vi "Main Page.vi"(8 "error in (no error)":errorcluster, 11 "Node Ptr":T1 format="%.0x") -> (0 "error out":errorcluster)   [LabVIEW 2019, in "DeltaPSControl System Explorer.lvlib"]
uses:
  DeltaPSControl System Explorer.lvlib
  <vilib>/NI VeriStand/Custom Device API/Custom Device Item Ref.ctl
  Shared/Constants.vi
  <vilib>/NI VeriStand/Custom Device API/Get Item Property (String).vi
  <vilib>/NI VeriStand/Custom Device API/Get Item Property (U16).vi
  <vilib>/NI VeriStand/Custom Device API/Get Item Property (String Array).vi
  <vilib>/NI VeriStand/Custom Device API/Set Item Property (String).vi
  <vilib>/NI VeriStand/Custom Device API/Set Item Property (U16).vi
  <vilib>/NI VeriStand/Custom Device API/Set Item Property (String Array).vi
  <vilib>/NI VeriStand/Custom Device API/Custom Device API.lvlib
  Shared/DeltaPSControl Shared.lvlib
panel:
  in  "Help":bool
  out "Sequences List":string[][](array[string])
  in  "LOAD Seq":bool
  in  "Port":u16
  in  "IP Address":string
  in  "Header":cluster{"Section Name":string}={"Section Name"="Custom Device Item Settings"}
  in  "Description":string
  in  "Name":string
  # "Always need to load\n sequences,\n to be able to use them."
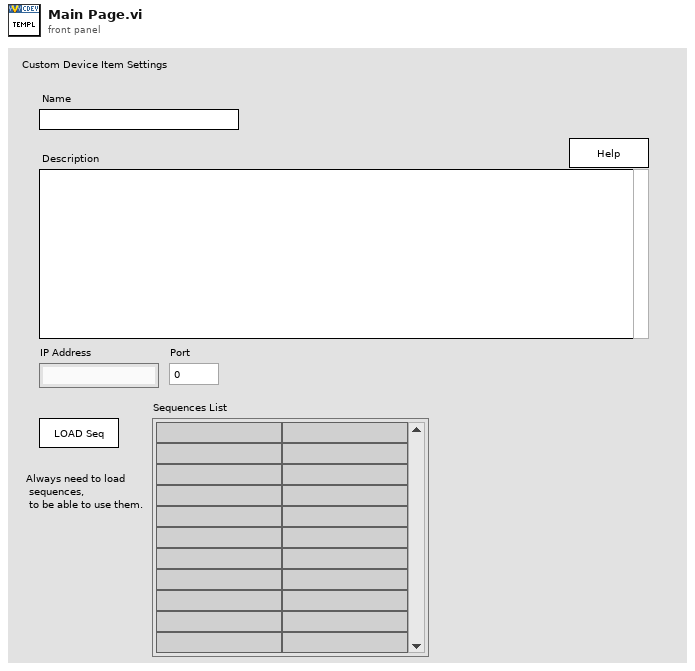
[diagram p1: front panel]
types:
  T1 = typedef "Custom Device API.lvlib/Custom Device Item Ref.ctl" = u64
  T2 = typedef "Custom Device API.lvlib/Custom Device Item Info.ctl" = cluster{"Name":string, "Is Channel":bool, "GUID":string, "Is Waveform":bool}
  T3 = typedef "Custom Device API.lvlib/Custom Device Commands.ctl" = enum16{"Default", "Item renamed", "Shutdown", "Dynamic button pressed"}
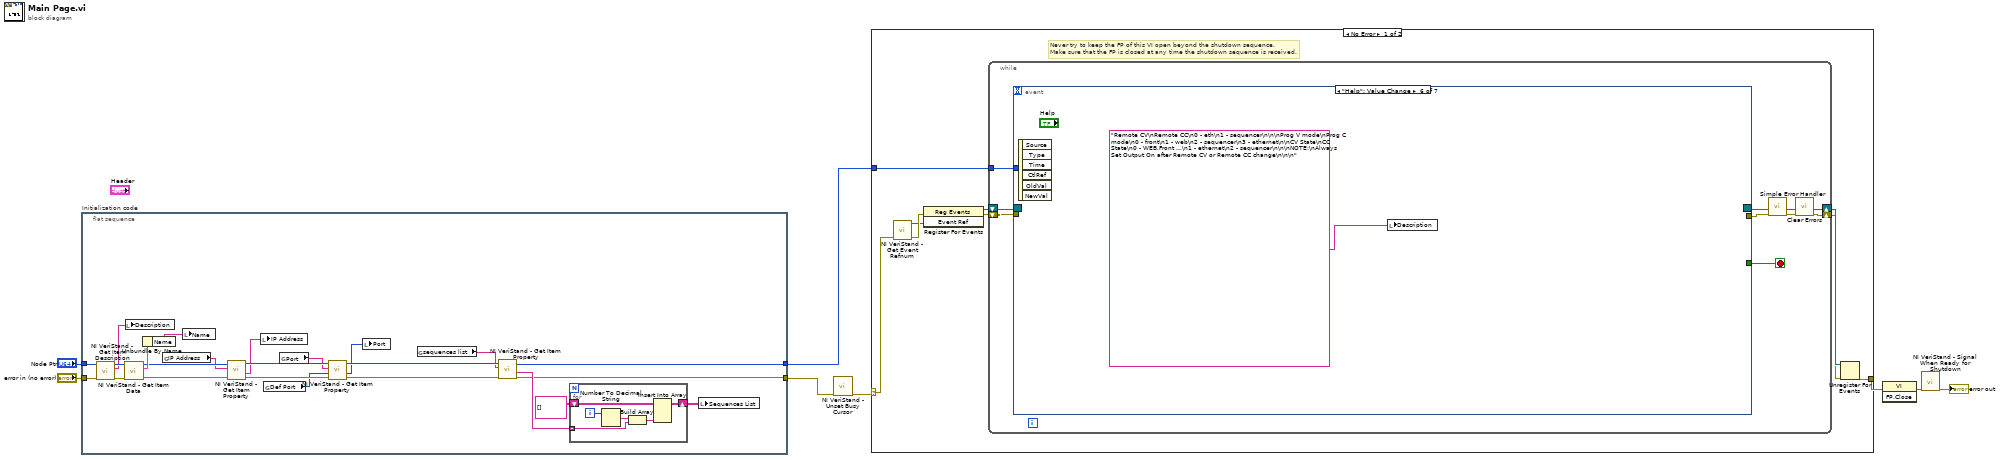
[diagram p0: block diagram]
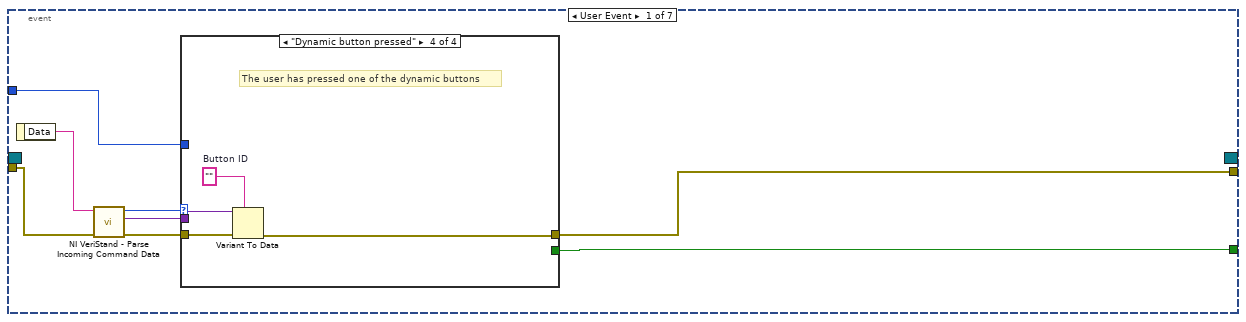
[diagram p2: hidden frame]
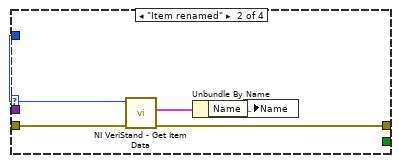
[diagram p4: hidden frame]
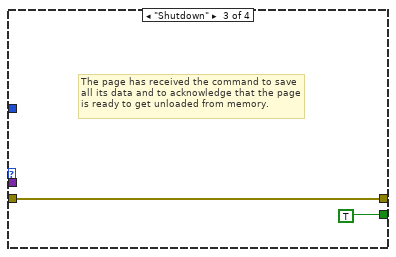
[diagram p5: hidden frame]
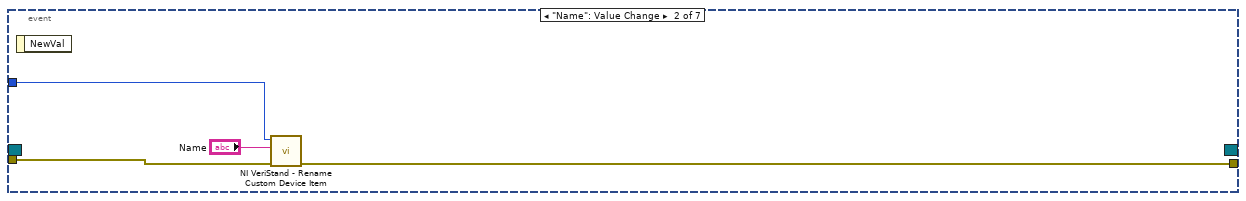
[diagram p6: hidden frame]
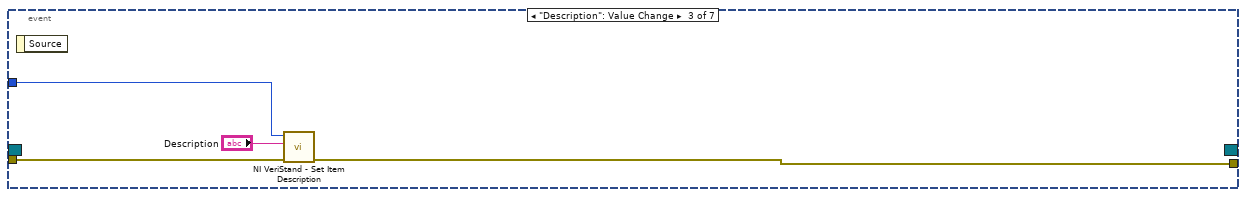
[diagram p7: hidden frame]
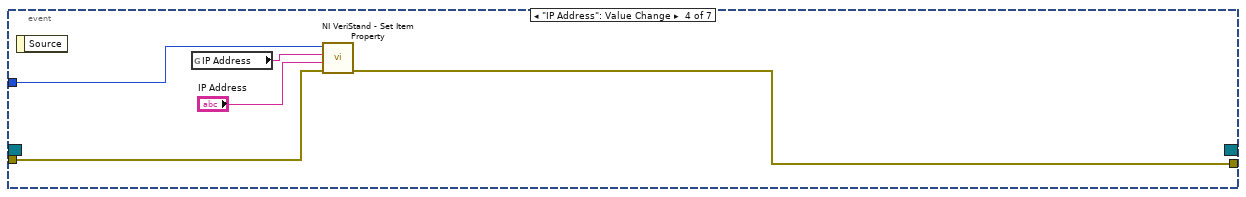
[diagram p8: hidden frame]
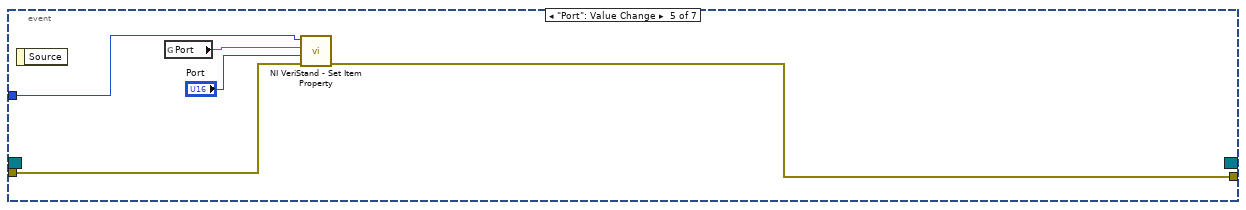
[diagram p9: hidden frame]
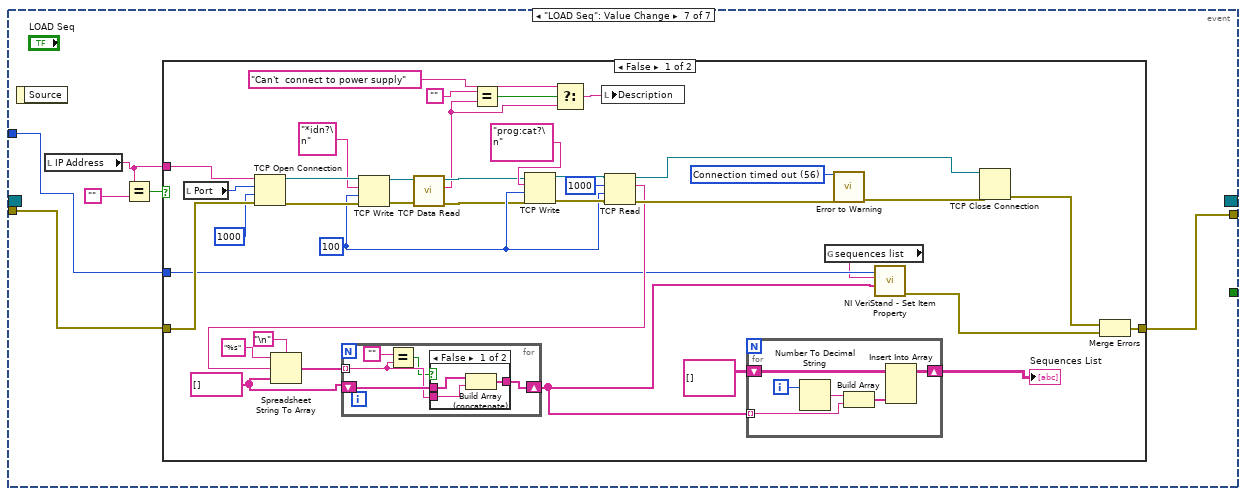
[diagram p10: hidden frame]
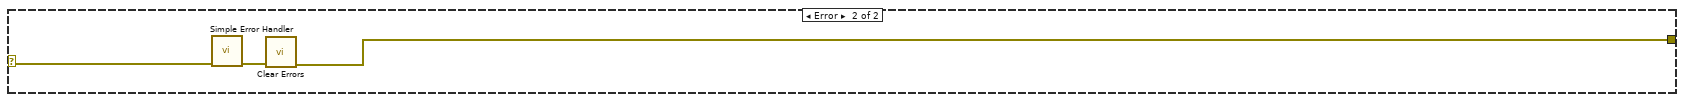
[diagram p13: hidden frame]
diagram:
  n1 = flat-sequence "Initialization code" {
    tunnel: "error in (no error)" -> [w31]
    tunnel: "Node Ptr" -> [w30]
    tunnel: [w16] -> w4
    tunnel: [w17] -> w1
    frame #0 {
      n2 = call <vilib>:"NI VeriStand - Get Item Description.vi"("error in (no error)"=w31, "Item Ref in"=w30) -> ("error out"=w28:errorcluster, "Description"=w29:string, "Item Ref out"=w32:T1)  [unwired: 7 out]
      n3 = call <vilib>:"NI VeriStand - Get Item Data.vi"("error in (no error)"=w28, "Item Ref in"=w32) -> ("error out"=w18:errorcluster, "Item Info"=w27:T2, "Item Ref out"=w19:T1)  [unwired: 7 out]
      n4 = local write "Description"(w29) -> ()
      n5 = Unbundle By Name(w27) -> ("Name"=w26:string)
      n6 = global read "Constants.vi" "IP Address"() -> (w12:string)
      n7 = local write "Name"(w26) -> ()
      n8 = call-poly <vilib>:"NI VeriStand - Get Item Property.vi"("error in (no error)"=w18, "Property Name"=w12, "Item Ref in"=w19) -> ("error out"=w21:errorcluster, "Value"=w15:string, "Item Ref out"=w22:T1)  [unwired: 5 in, 1 out]
      n9 = local write "IP Address"(w15) -> ()
      n10 = global read "Constants.vi" "Def Port"() -> (w9:u16)
      n11 = global read "Constants.vi" "Port"() -> (w11:string)
      n12 = call-poly <vilib>:"NI VeriStand - Get Item Property.vi"("error in (no error)"=w21, "Default Value"=w9, "Property Name"=w11, "Item Ref in"=w22) -> ("error out"=w23:errorcluster, "Value"=w14:u16, "Item Ref out"=w24:T1)  [unwired: 4 in, 1 out]
      n13 = local write "Port"(w14) -> ()
      n14 = global read "Constants.vi" "sequences list"() -> (w10:string)
      n15 = call-poly <vilib>:"NI VeriStand - Get Item Property.vi"("error in (no error)"=w23, "Property Name"=w10, "Item Ref in"=w24) -> ("error out"=w16:errorcluster, "Value"=w25:string[], "Item Ref out"=w17:T1)  [unwired: 5 in, 1 out]
      n16 = for {
        shift-right: [w37] -> w13
        shift-left: string[][] [] -> [w38]
        tunnel: w25 -> [w33] mode=indexing
        i -> [w36]
        n17 = Number To Decimal String(number=w36) -> (decimal integer string=w35:string)  [unwired: 1 in]
        n18 = Build Array(w35, w33) -> (w34:string[])
        n19 = Insert Into Array(array=w38, new element=w34) -> (w37:string[][])  [unwired: 2 in]
      }
      n20 = local write "Sequences List"(w13) -> ()
    }
  }
  n21 = call <vilib>:"NI VeriStand - Unset Busy Cursor.vi"("error in (no error)"=w4) -> ("error out"=w3:errorcluster)  [unwired: 10 out]
  n22 = case shown="No Error" w3 {
    selector: w3 -> [w39 w157]
    tunnel: [w44 w155] -> w8
    tunnel: w1 -> [w40 _]
    frame No Error {
      # "Never try to keep the FP of this VI open beyond the shutdown sequence.\nMake sure that the FP is closed at any time the shutdown sequence is received."
      n23 = call <vilib>:"NI VeriStand - Get Event Refnum.vi"("error in (no error)"=w39) -> ("error out"=w47:errorcluster, "Event Ref"=w43:refnum<user-event>)  [unwired: 9 out]
      n24 = register-events(error in=w47, w43) -> (reference out=w41:refnum<event-registration>, error out=w42:errorcluster)  [unwired: 1 in]
      n25 = while {
        tunnel: w40 -> [w51]
        shift-right: [w48] -> w45
        shift-left: w42 -> [w54]
        shift-right: [w55] -> w46
        shift-left: w41 -> [w53]
        stop <- w52 stop-if-true
        n26 = event shown="[5] \"Help\": Value Change" {
          selector: w53 -> [_ _ _ _ _ _ _]
          dyn-events: [_ _ _ _ _ _ _] -> w55
          timeout: _ -> [_ _ _ _ _ _ _]
          tunnel: w54 -> [w63 w79 w82 w86 w92 _ w96]
          tunnel: [w59 _ _ _ _ _ _] -> w52
          tunnel: [w58 w78 w81 w85 w91 _ w95] -> w50
          tunnel: w51 -> [w57 w77 w83 w87 w89 _ w97]
          event User Event {
            n27 = event-data() -> ("Data"=w62:string)  [unwired: 1 out]
            n28 = call <vilib>:"NI VeriStand - Parse Incoming Command Data.vi"("error in (no error)"=w63, "Incoming data"=w62) -> ("error out"=w61:errorcluster, "Outgoing data"=w56:variant, "Action"=w60:T3)  [unwired: 7 out]
            n29 = case shown="\"Dynamic button pressed\"" w60 {
              tunnel: w61 -> [w64 w69 w70 w75]
              tunnel: [_ _ TRUE _] -> w59
              tunnel: [w64 w66 w70 w72] -> w58
              tunnel: w57 -> [_ w68 _ _]
              tunnel: w56 -> [_ _ _ w74]
              frame "Default", Default {
              }
              frame "Item renamed" {
                n30 = call <vilib>:"NI VeriStand - Get Item Data.vi"("error in (no error)"=w69, "Item Ref in"=w68) -> ("error out"=w66:errorcluster, "Item Info"=w67:T2)  [unwired: 8 out]
                n31 = Unbundle By Name(w67) -> ("Name"=w65:string)
                n32 = local write "Name"(w65) -> ()
              }
              frame "Shutdown" {
                # "The page has received the command to save all its data and to acknowledge that the page is ready to get unloaded from memory."
              }
              frame "Dynamic button pressed" {
                w73 = ""  # Button ID
                # "The user has pressed one of the dynamic buttons"
                n33 = Variant To Data(error in=w75, type=w73, Variant=w74) -> (error out=w72:errorcluster)  [unwired: 1 out]
              }
            }
          }
          event "Name": Value Change {
            n34 = event-data() -> ()  [unwired: 2 out]
            n35 = call <vilib>:"NI VeriStand - Rename Custom Device Item.vi"("error in (no error)"=w79, "New Name"="Name", "Item Ref in"=w77) -> ("error out"=w78:errorcluster)  [unwired: 1 in, 7 out]
          }
          event "Description": Value Change {
            n36 = event-data() -> ()  [unwired: 2 out]
            n37 = call <vilib>:"NI VeriStand - Set Item Description.vi"("error in (no error)"=w82, "Description"="Description", "Item Ref in"=w83) -> ("error out"=w81:errorcluster)  [unwired: 8 out]
          }
          event "IP Address": Value Change {
            n38 = event-data() -> ()  [unwired: 2 out]
            n39 = global read "Constants.vi" "IP Address"() -> (w88:string)
            n40 = call-poly <vilib>:"NI VeriStand - Set Item Property.vi"("error in (no error)"=w86, "Value"="IP Address", "Property Name"=w88, "Item Ref in"=w87) -> ("error out"=w85:errorcluster)  [unwired: 5 in, 2 out]
          }
          event "Port": Value Change {
            n41 = event-data() -> ()  [unwired: 2 out]
            n42 = global read "Constants.vi" "Port"() -> (w90:string)
            n43 = call-poly <vilib>:"NI VeriStand - Set Item Property.vi"("error in (no error)"=w92, "Value"="Port", "Property Name"=w90, "Item Ref in"=w89) -> ("error out"=w91:errorcluster)  [unwired: 5 in, 2 out]
          }
          event "Help": Value Change {
            n44 = event-data() -> ()  [unwired: 7 out]
            n45 = local write "Description"("Remote CV\nRemote CC\n0 - eth\n1 - sequencer\n\n\nProg V mode\nProg C mode\n0 - front\n1 - web\n2 - sequencer\n3 - ethernet\n\nCV State\nCC State\n0 - WEB,Front ...\n1 - ethernet\n2 - sequencer\n\n\nNOTE:\nAlways Set Output On after Remote CV or Remote CC change\n\n\n") -> ()
          }
          event "LOAD Seq": Value Change {
            n46 = event-data() -> ()  [unwired: 2 out]
            n47 = local read "IP Address"() -> (w98:string)
            n48 = Equal?(x=w98, y="") -> (x = y?=w99:bool)
            n49 = case shown="False" w99 {
              tunnel: w96 -> [w138 w154]
              tunnel: w98 -> [w137 _]
              tunnel: [w119 w154] -> w95
              tunnel: w97 -> [w118 _]
              frame False {
                w126 = string[] []
                w128 = 56 items=["No Error", "Argument Error", "Memory Full", "Out of Zone", "End of File", "File Already Open", "Generic File IO Error", "File Not Found", "File Permission Error", "Disk Full", "Duplicate Path", "Too Many Files Open", "Not Enabled", "Resource File Not Found", "Cannot Add Resource", "Resource Not Found", "Image Not Found", "Image Memory Error", "Pen Does Not Exist", "Config Bad Type", "Config Token Not Found", "Config Parse Error", "Config Memory Error", "Bad External Code Format", "Bad External Code Offset", "External Code Not Present", "Null Window", "Destroy Window Mixup", "Null Menu", "Print Aborted", "Bad Print Record", "Print Driver Error", "Windows Error During Print", "Memory Error During Print", "Print Dialog Error", "Generic Print Error", "Invalid Device Refnum", "Device Not Found", "Device Parameter Error", "Device Unit Error", "Can't Open Device", "Device Call Aborted", "Generic Error", "Cancelled By User", "Object ID Too Low", "Object ID Too High", "Object Not In Heap", "Unknown Heap", "Bad DefProc ID", "DefProc Not In Table", "Message Out Of Range", "Null Method", "Unknown Message", "Manager Call Not Supported", "Bad address", "Connection In progress", "Connection timed out", "Connection is already in progress", "Network attribute not supported", "Network error", "Address in use", "System out of memory", "Connection aborted", "Connection refused", "Connection is not connected", "Connection is already connected", "Connection closed", "Initialize error (interapplication manager)", "Bad occurrence", "Wait on unbound occurrence handler", "Occurrence queue overflow", "Bad path", "Semaphore not signaled", "Unrecognized type (interapplication manager)"] ("1st Error to Convert")
                w130 = 100 ("timeout ms (25000)")
                n50 = local read "Port"() -> (w108:u16)
                n51 = TCP Open Connection(address=w137, remote port or service name=w108, timeout ms (60000)=1000, error in (no error)=w138) -> (connection ID=w136:refnum<k5>, error out=w135:errorcluster)  [unwired: 1 in]
                n52 = TCP Write(connection ID=w136, data in="*idn?\n", error in (no error)=w135, 9:w130) -> (connection ID out=w107:refnum<k5>, error out=w106:errorcluster)  [unwired: 1 out]
                n53 = call "TCP Data Read.vi"("error in (no error)"=w106, "Connection ID in"=w107) -> ("error out"=w104:errorcluster, "TCP Read data"=w103:string, "Connection ID out"=w105:refnum<k5>)  [unwired: 6 in, 1 out]
                n54 = Equal?(x="", y=w103) -> (x = y?=w111:bool)
                n55 = TCP Write(connection ID=w105, data in="prog:cat?\n", error in (no error)=w104, 9:w130) -> (connection ID out=w133:refnum<k5>, error out=w132:errorcluster)  [unwired: 1 out]
                n56 = Select(t="Can't  connect to power supply", s=w111, f=w103) -> (s? t:f=w109:string)
                n57 = local write "Description"(w109) -> ()
                n58 = TCP Read(connection ID=w133, bytes to read=1000, error in (no error)=w132, 9:w130) -> (connection ID out=w122:refnum<k5>, data out=w123:string, error out=w129:errorcluster)  [unwired: 1 in]
                n59 = Spreadsheet String To Array(delimiter (Tab)="\n", format string="%s", spreadsheet string=w123, array type (2D Dbl)=w126) -> (array=w127:string[])
                n60 = for {
                  tunnel: w127 -> [w147] mode=indexing
                  shift-right: [w148] -> w114
                  shift-left: w126 -> [w149]
                  n61 = Equal?(x="", y=w147) -> (x = y?=w145:bool)
                  n62 = case shown="False" w145 {
                    tunnel: w149 -> [w152 w153]
                    tunnel: w147 -> [w151 _]
                    tunnel: [w150 w153] -> w148
                    frame False {
                      n63 = Build Array (concatenate)(w152, w151) -> (w150:string[])
                    }
                    frame True {
                    }
                  }
                }
                n64 = for {
                  shift-right: [w143] -> w102
                  shift-left: string[][] [] -> [w144]
                  tunnel: w114 -> [w139] mode=indexing
                  i -> [w142]
                  n65 = Number To Decimal String(number=w142) -> (decimal integer string=w141:string)  [unwired: 1 in]
                  n66 = Build Array(w141, w139) -> (w140:string[])
                  n67 = Insert Into Array(array=w144, new element=w140) -> (w143:string[][])  [unwired: 2 in]
                }
                "Sequences List" <- w102
                n68 = global read "Constants.vi" "sequences list"() -> (w101:string)
                n69 = call <vilib>:"Error to Warning.vi"("1st Error to Convert"=w128, "error in"=w129) -> ("warning out"=w121:errorcluster)  [unwired: 13 in]
                n70 = call-poly <vilib>:"NI VeriStand - Set Item Property.vi"("Value"=w114, "Property Name"=w101, "Item Ref in"=w118) -> ("error out"=w116:errorcluster)  [unwired: 6 in, 2 out]
                n71 = TCP Close Connection(connection ID=w122, error in (no error)=w121) -> (error out=w120:errorcluster)  [unwired: 1 in, 1 out]
                n72 = Merge Errors(w120, w116) -> (w119:errorcluster)
              }
              frame True {
                # "EMPTY"
              }
            }
          }
        }
        n73 = call <vilib>:"Simple Error Handler.vi"("error in (no error)"=w50) -> ("error out"=w49:errorcluster)  [unwired: 1 in, 7 out]
        n74 = call <vilib>:"Clear Errors.vi"("error in (no error)"=w49) -> ("error out"=w48:errorcluster)  [unwired: 1 in, 5 out]
      }
      n75 = Unregister For Events(event registration refnum=w46, error in=w45) -> (error out=w44:errorcluster)
    }
    frame Error {
      n76 = call <vilib>:"Simple Error Handler.vi"("error in (no error)"=w157) -> ("error out"=w156:errorcluster)  [unwired: 1 in, 7 out]
      n77 = call <vilib>:"Clear Errors.vi"("error in (no error)"=w156) -> ("error out"=w155:errorcluster)  [unwired: 1 in, 5 out]
    }
  }
  n78 = invoke class="VI" method="FP.Close"(error in=w8) -> (error out=w7:errorcluster)  [unwired: 2 in, 2 out]
  n79 = call <vilib>:"NI VeriStand - Signal When Ready for Shutdown.vi"("error in (no error)"=w7) -> ("error out"=→"error out":errorcluster)  [unwired: 10 out]
